vi "Apply Range Color.vi"(4 "Range":dbl, 6 "Ideal":dbl, 8 "error in (no error)":errorcluster, 9 "Value":dbl, 11 "GaugeIndicator in":refnum<class "GaugeIndicator.lvclass">) -> (0 "error out":errorcluster, 3 "GaugeIndicator out":refnum<class "GaugeIndicator.lvclass">)   [LabVIEW 2020, in "VolatusGUIElements.lvlib" / "GaugeIndicator.lvclass"]
uses:
  GaugeIndicator.lvclass
  GaugeIndicator.lvclass/GaugeIndicator.ctl
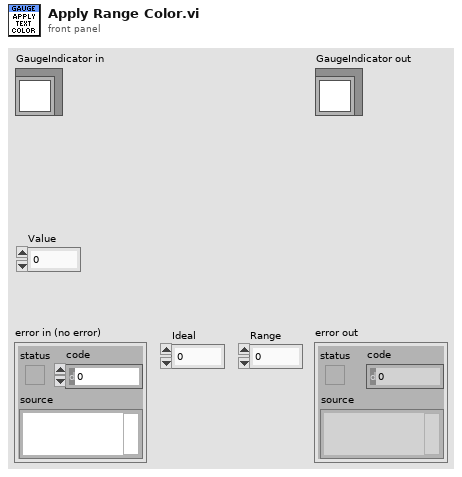
[diagram p1: front panel]
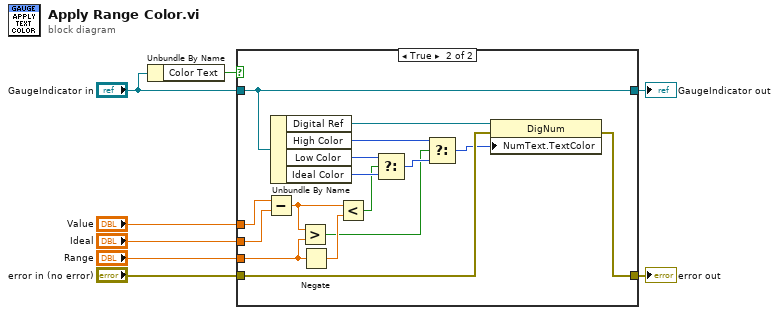
[diagram p0: block diagram]
diagram:
  n1 = Unbundle By Name("GaugeIndicator in") -> ("Color Text"=w8:bool)
  n2 = case shown="True" w8 {
    tunnel: [w10 w11] -> w7
    tunnel: "GaugeIndicator in" -> [w10 w11]
    tunnel: "error in (no error)" -> [w9 w26]
    tunnel: [w9 w12] -> w4
    tunnel: "Value" -> [_ w24]
    tunnel: "Ideal" -> [_ w23]
    tunnel: "Range" -> [_ w22]
    frame False {
    }
    frame True {
      n3 = Subtract(x=w24, y=w23) -> (x-y=w21:dbl)
      n4 = Unbundle By Name(w11) -> ("Digital Ref"=w25:refnum<vi>, "High Color"=w16:u32, "Low Color"=w18:u32, "Ideal Color"=w19:u32)
      n5 = Greater?(x=w21, y=w22) -> (0:w14:bool)
      n6 = Negate(x=w22) -> (-x=w20:dbl)
      n7 = Less?(x=w21, y=w20) -> (x < y?=w17:bool)
      n8 = Select(t=w18, s=w17, f=w19) -> (s? t:f=w15:u32)
      n9 = Select(t=w16, s=w14, f=w15) -> (s? t:f=w13:u32)
      n10 = property class="DigNum"(reference=w25, error in=w26, "NumText.TextColor"=w13) -> (error out=w12:errorcluster)  [unwired: 1 out]
    }
  }
  "error out" <- w4
  "GaugeIndicator out" <- w7
